vi "Auton - Boiler Gear.vi"(10 "Alliance":T2, 11 "Auton States":T1=enum."Reset Encoders") -> ()   [LabVIEW 2016]
uses:
  Auton - Boiler Gear States.ctl
  <vilib>/Rock Robotics/WPI/DriverStation/WPI_DriverStationAllianceInfo.ctl
panel:
  out "Current State":T1
  in  "Drive Forward to Peg with Vision":dbl=50.0
  in  "Mount Peg Distance SP":dbl=15.0
  in  "Turn Adjust Blue":dbl=58.0
  in  "Turn Adjust Red":dbl=302.0
  in  "Back Away SP":dbl
  in  "Red - Face Airship Setpoint":dbl=286.0
  in  "Blue - Face Airship Setpoint":dbl=74.0
  in  "Drive Forward Set Point":dbl=72.0
  # "76"
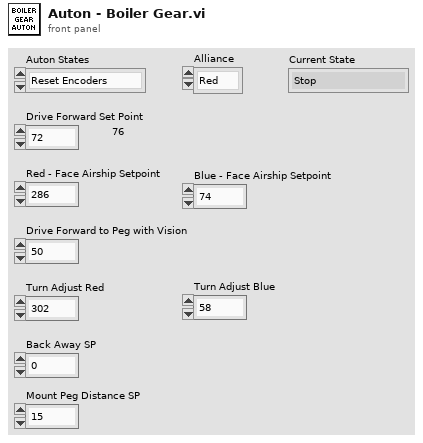
[diagram p1: front panel]
types:
  T1 = typedef "Auton - Boiler Gear States.ctl" = enum16{"Stop", "Reset Encoders", "Drive Forward", "Face Airship Gyro", "Reset Encoders Again", "Drive Forward to Peg", "Turn to Mount Peg", "Mount Peg", "Eject Gear", "Back Away", "Reset Encoders Again Again"}
  T2 = typedef "WPI_DriverStationAllianceInfo.ctl" = enum16{"Red", "Blue", "Invalid"}
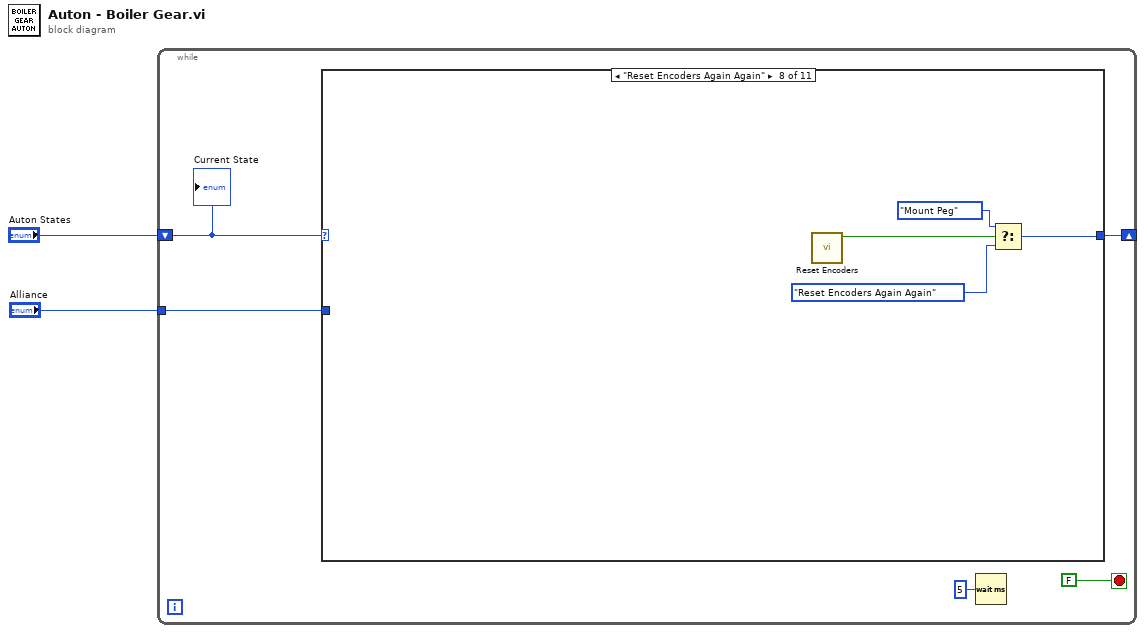
[diagram p0: block diagram]
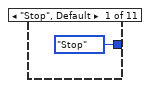
[diagram p2: hidden frame]
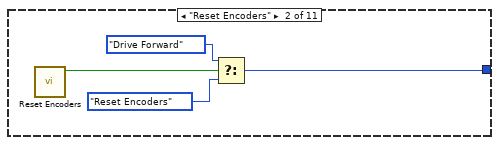
[diagram p3: hidden frame]
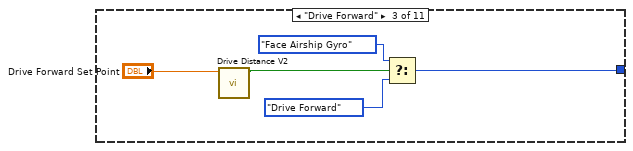
[diagram p4: hidden frame]
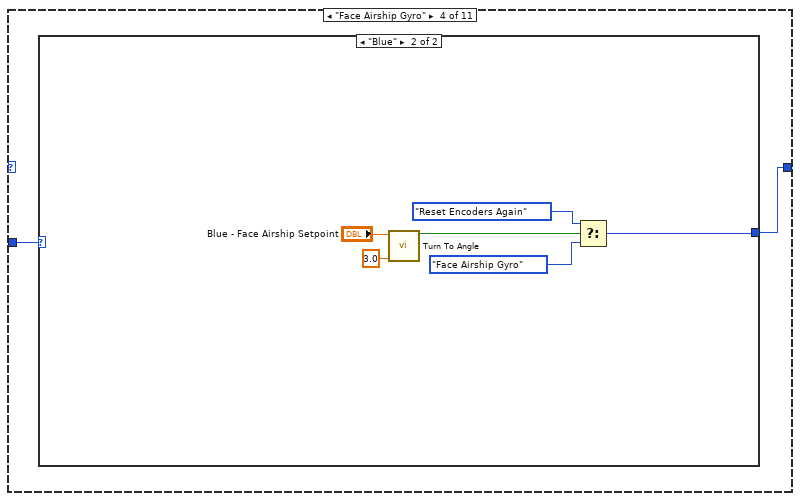
[diagram p5: hidden frame]
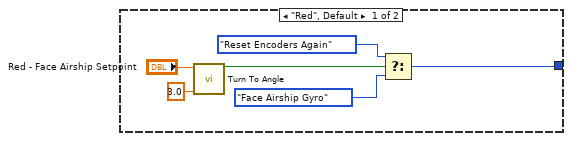
[diagram p6: hidden frame]
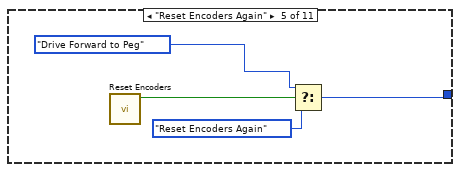
[diagram p7: hidden frame]
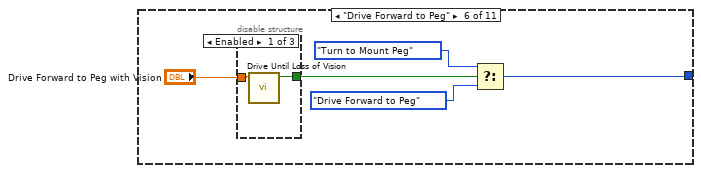
[diagram p8: hidden frame]
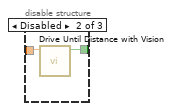
[diagram p9: hidden frame]
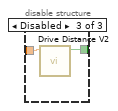
[diagram p10: hidden frame]
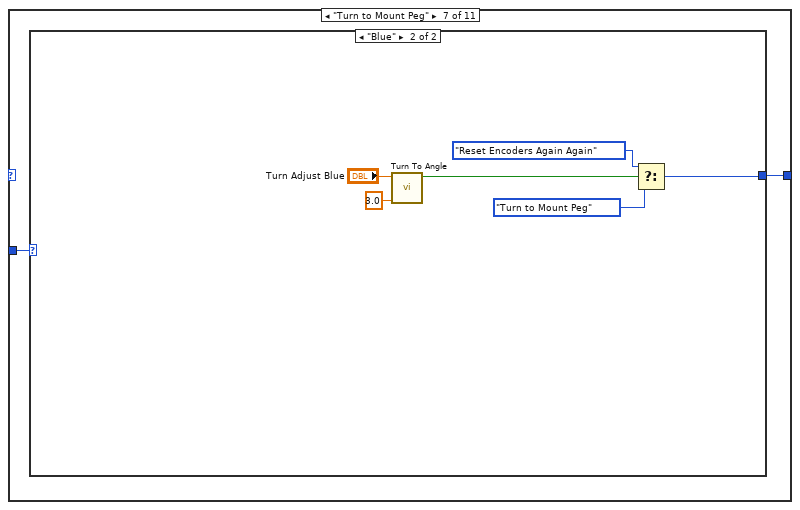
[diagram p11: hidden frame]
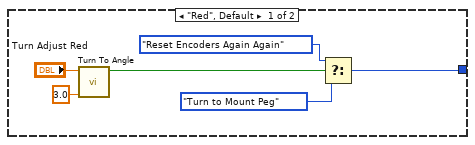
[diagram p12: hidden frame]
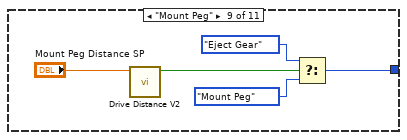
[diagram p13: hidden frame]
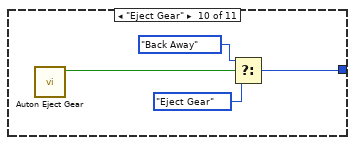
[diagram p14: hidden frame]
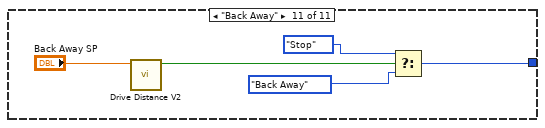
[diagram p15: hidden frame]
diagram:
  n1 = while {
    tunnel: "Alliance" -> [w7]
    shift-right: [w4] -> _
    shift-left: "Auton States" -> [w5]
    stop <- FALSE stop-if-true
    n2 = case shown="\"Reset Encoders Again Again\"" w5 {
      tunnel: w7 -> [_ _ _ w19 _ _ w47 _ _ _ _]
      tunnel: [Auton_-_Boiler_Gear_States."Stop" ("f") w10 w14 w18 w33 w39 w48 w61 w65 w71 w76] -> w4
      frame "Stop", Default {
      }
      frame "Reset Encoders" {
        n3 = call "Reset Encoders.vi"() -> ("Done?"=w12:bool)  [unwired: 11 in]
        n4 = Select(t=Auton_-_Boiler_Gear_States."Drive Forward" ("Auton States"), s=w12, f=Auton_-_Boiler_Gear_States."Reset Encoders") -> (s? t:f=w10:T1)
      }
      frame "Drive Forward" {
        n5 = call "Drive Distance V2.vi"("Distance Set Point"="Drive Forward Set Point") -> ("Done?"=w15:bool)  [unwired: 10 in]
        n6 = Select(t=Auton_-_Boiler_Gear_States."Face Airship Gyro" ("Auton States"), s=w15, f=Auton_-_Boiler_Gear_States."Drive Forward") -> (s? t:f=w14:T1)
      }
      frame "Face Airship Gyro" {
        n7 = case shown="\"Blue\"" w19 {
          tunnel: [w21 w27] -> w18
          frame "Red", Default {
            n8 = call "Turn To Angle.vi"("Turn Angle Tolerance"=3.0, "Setpoint"="Red - Face Airship Setpoint") -> ("Done?"=w25:bool)  [unwired: 9 in]
            n9 = Select(t=Auton_-_Boiler_Gear_States."Reset Encoders Again" ("Auton States"), s=w25, f=Auton_-_Boiler_Gear_States."Face Airship Gyro") -> (s? t:f=w21:T1)
          }
          frame "Blue" {
            n10 = call "Turn To Angle.vi"("Turn Angle Tolerance"=3.0, "Setpoint"="Blue - Face Airship Setpoint") -> ("Done?"=w28:bool)  [unwired: 9 in]
            n11 = Select(t=Auton_-_Boiler_Gear_States."Reset Encoders Again" ("Auton States"), s=w28, f=Auton_-_Boiler_Gear_States."Face Airship Gyro") -> (s? t:f=w27:T1)
          }
        }
      }
      frame "Reset Encoders Again" {
        n12 = call "Reset Encoders.vi"() -> ("Done?"=w34:bool)  [unwired: 11 in]
        n13 = Select(t=Auton_-_Boiler_Gear_States."Drive Forward to Peg" ("Auton States"), s=w34, f=Auton_-_Boiler_Gear_States."Reset Encoders Again") -> (s? t:f=w33:T1)
      }
      frame "Drive Forward to Peg" {
        n14 = disable-structure shown="Enabled" {
          disable-tunnel: [w42 w44 w45] -> w37
          disable-tunnel: "Drive Forward to Peg with Vision" -> [w41 w43 w46]
          frame Enabled {
            n15 = call "Drive Until Loss of Vision.vi"("Distance Setpoint"=w41) -> ("ready to approach"=w42:bool)  [unwired: 10 in]
          }
          frame Disabled {
            n16 = call "Drive Until Distance with Vision.vi"("Distance Set Point"=w43) -> ("Done?"=w44:bool)  [unwired: 10 in]
          }
          frame Disabled {
            n17 = call "Drive Distance V2.vi"("Distance Set Point"=w46) -> ("Done?"=w45:bool)  [unwired: 10 in]
          }
        }
        n18 = Select(t=Auton_-_Boiler_Gear_States."Turn to Mount Peg" ("Auton States"), s=w37, f=Auton_-_Boiler_Gear_States."Drive Forward to Peg" ("Auton States")) -> (s? t:f=w39:T1)
      }
      frame "Turn to Mount Peg" {
        n19 = case shown="\"Blue\"" w47 {
          tunnel: [w51 w58] -> w48
          frame "Red", Default {
            n20 = call "Turn To Angle.vi"("Turn Angle Tolerance"=3.0, "Setpoint"="Turn Adjust Red") -> ("Done?"=w54:bool)  [unwired: 9 in]
            n21 = Select(t=Auton_-_Boiler_Gear_States."Reset Encoders Again Again" ("Auton States"), s=w54, f=Auton_-_Boiler_Gear_States."Turn to Mount Peg") -> (s? t:f=w51:T1)
          }
          frame "Blue" {
            n22 = call "Turn To Angle.vi"("Turn Angle Tolerance"=3.0, "Setpoint"="Turn Adjust Blue") -> ("Done?"=w57:bool)  [unwired: 9 in]
            n23 = Select(t=Auton_-_Boiler_Gear_States."Reset Encoders Again Again" ("Auton States"), s=w57, f=Auton_-_Boiler_Gear_States."Turn to Mount Peg") -> (s? t:f=w58:T1)
          }
        }
      }
      frame "Reset Encoders Again Again" {
        n24 = call "Reset Encoders.vi"() -> ("Done?"=w64:bool)  [unwired: 11 in]
        n25 = Select(t=Auton_-_Boiler_Gear_States."Mount Peg" ("Auton States"), s=w64, f=Auton_-_Boiler_Gear_States."Reset Encoders Again Again") -> (s? t:f=w61:T1)
      }
      frame "Mount Peg" {
        n26 = call "Drive Distance V2.vi"("Distance Set Point"="Mount Peg Distance SP") -> ("Done?"=w66:bool)  [unwired: 10 in]
        n27 = Select(t=Auton_-_Boiler_Gear_States."Eject Gear" ("f"), s=w66, f=Auton_-_Boiler_Gear_States."Mount Peg") -> (s? t:f=w65:T1)
      }
      frame "Eject Gear" {
        n28 = call "Auton Eject Gear.vi"() -> ("Done?"=w70:bool)  [unwired: 11 in]
        n29 = Select(t=Auton_-_Boiler_Gear_States."Back Away" ("Auton States"), s=w70, f=Auton_-_Boiler_Gear_States."Eject Gear") -> (s? t:f=w71:T1)
      }
      frame "Back Away" {
        n30 = call "Drive Distance V2.vi"("Distance Set Point"="Back Away SP") -> ("Done?"=w77:bool)  [unwired: 10 in]
        n31 = Select(t=Auton_-_Boiler_Gear_States."Stop" ("Auton States"), s=w77, f=Auton_-_Boiler_Gear_States."Back Away" ("Auton States")) -> (s? t:f=w76:T1)
      }
    }
    n32 = Wait (ms)(milliseconds to wait=u32 5) -> ()  [unwired: 1 out]
    "Current State" <- w5
  }
